vi "CreateCesTML.vi"(8 "error in (no error)":errorcluster, 10 "Traffic String":string="{\"longitude\":-79.645,\"latitude\":39.75710,\"height\":30000,\"ICAO\":\"AAAA\"},{\"longitude\":-79.645,\"latitude\":39.75710,\"height\":5000,\"ICAO\":\"BBBB\"}", 11 "ViewerData":T1={"ViewerLat"="40.286792", "ViewerLong"="-79.541260", "ViewerAlt"="1000", "ViewerHDG"="270", "Viewerpitch"="0"}) -> (0 "error out":errorcluster)   [LabVIEW 2020]
uses:
  <vilib>/Utility/NIReport.llb/Report Type.ctl
  <vilib>/printing/OpenHTMLReport.llb/Open HTML Report in Browser (Refnum).vi
  <vilib>/Utility/NIReport.llb/NI_report.lvclass
  <vilib>/Utility/NIReport.llb/NI_ReportGenerationCore.lvlib
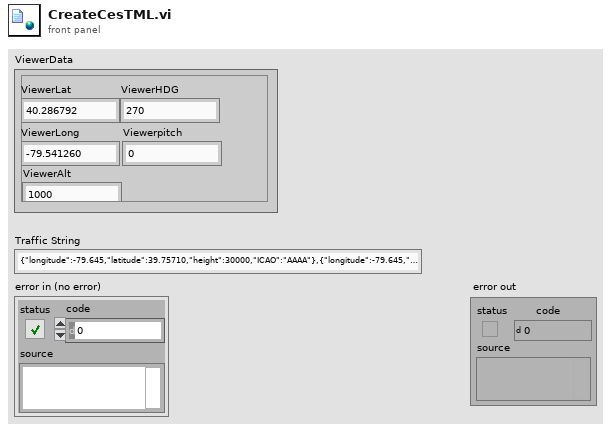
[diagram p1: front panel]
types:
  T1 = cluster{"ViewerLat":string, "ViewerLong":string, "ViewerAlt":string, "ViewerHDG":string, "Viewerpitch":string}
  T2 = typedef "NI_ReportGenerationCore.lvlib/Report Type.ctl" = enum16{"HTML", "Word", "Excel"}
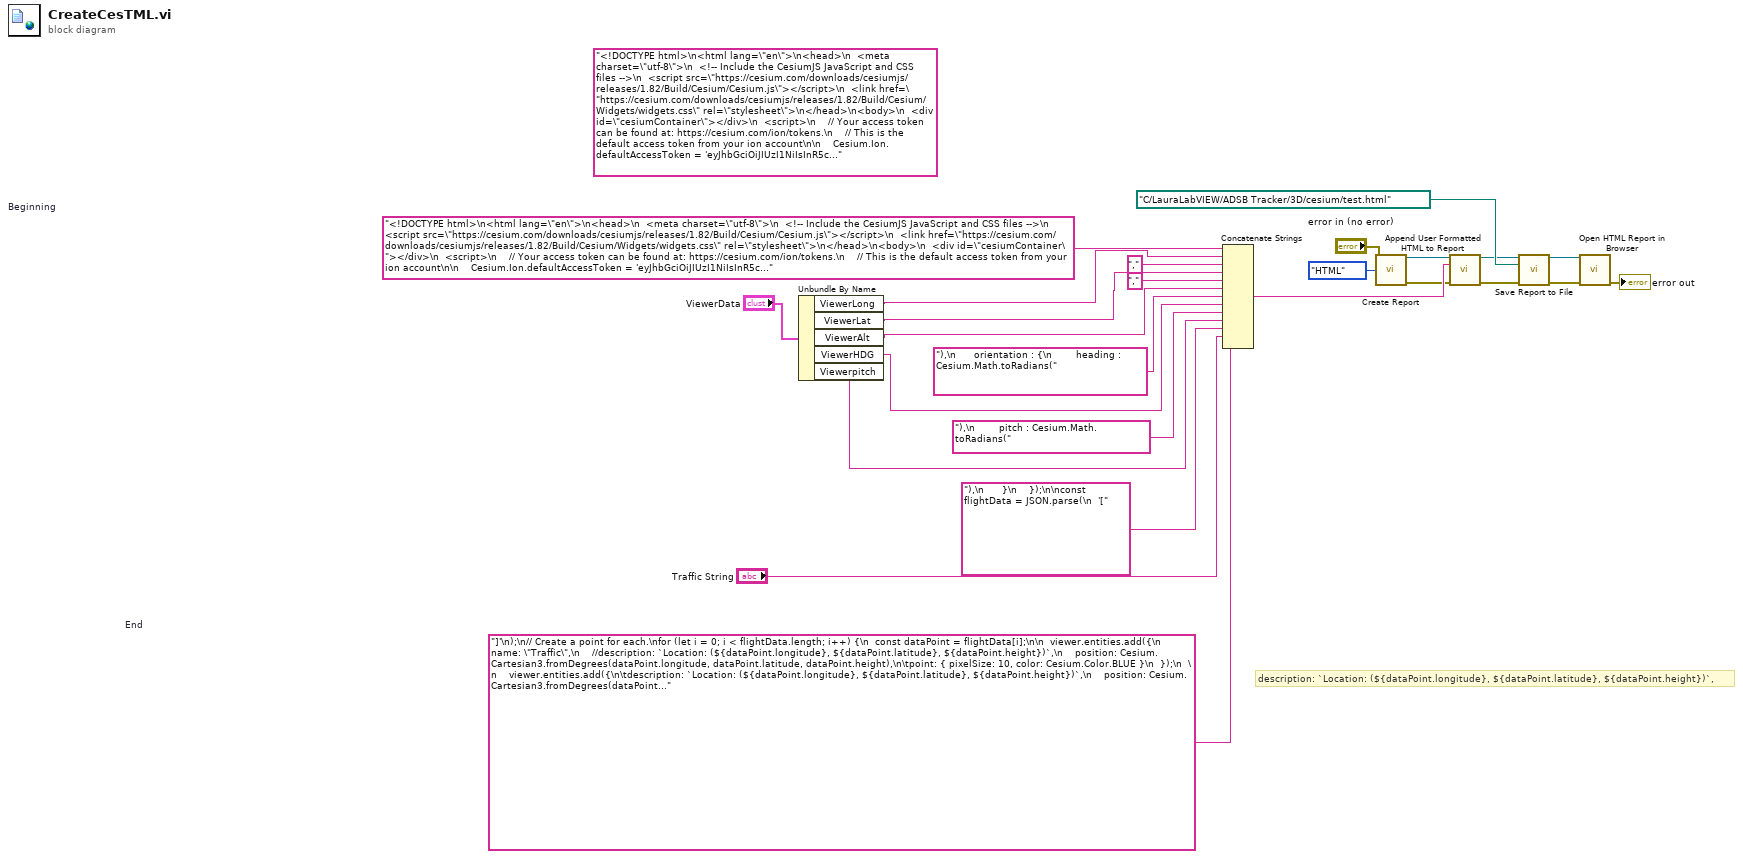
[diagram p0: block diagram]
diagram:
  (unwired) "<!DOCTYPE html>\n<html lang=\"en\">\n<head>\n  <meta charset=\"utf-8\">\n  <!-- Include the CesiumJS JavaScript and CSS files -->\n  <script src=\"https://cesium.com/downloads/cesiumjs/releases/1.82/Build/Cesium/Cesium.js\"></script>\n  <link href=\"https://cesium.com/downloads/cesiumjs/releases/1.82/Build/Cesium/Widgets/widgets.css\" rel=\"stylesheet\">\n</head>\n<body>\n  <div id=\"cesiumContainer\"></div>\n  <script>\n    // Your access token can be found at: https://cesium.com/ion/tokens.\n    // This is the default access token from your ion account\n\n    Cesium.Ion.defaultAccessToken = 'eyJhbGciOiJIUzI1NiIsInR5cCI6IkpXVCJ9.eyJqdGkiOiJmZmNkNjRiZS1hOTkzLTRmNDYtOTM2Mi1iMTFiN2ZmOTk1NzAiLCJpZCI6NjAzMTEsImlhdCI6MTYyNDk3NjYyMX0.UAa42undAhoI0-5rRI83UHZD0L_t9PndA7YpwJBLA6o';\n\t\n\t  // Initialize the Cesium Viewer in the HTML element with the `cesiumContainer` ID.\n    const viewer = new Cesium.Viewer('cesiumContainer', {\n      terrainProvider: Cesium.createWorldTerrain()\n    });    \n    // Add Cesium OSM Buildings, a global 3D buildings layer.\n    const buildingTileset = viewer.scene.primitives.add(Cesium.createOsmBuildings());   \n    // Fly the camera to viewer location\n    viewer.camera.flyTo({\n      destination : Cesium.Cartesian3.fromDegrees(-122.4175, 37.655, 1000),\n      orientation : {\n        heading : Cesium.Math.toRadians(270),\n        pitch : Cesium.Math.toRadians(0),\n      }\n    });\n\nconst flightData = JSON.parse(\n  '[{\"longitude\":-122.39053,\"latitude\":37.61779,\"height\":-27.32},{\"longitude\":-122.39035,\"latitude\":37.61803,\"height\":-27.32}]'\n);\n// Create a point for each.\nfor (let i = 0; i < flightData.length; i++) {\n  const dataPoint = flightData[i];\n\n  viewer.entities.add({\n  name: \"Traffic\",\n    //description: `Location: (${dataPoint.longitude}, ${dataPoint.latitude}, ${dataPoint.height})`,\n    position: Cesium.Cartesian3.fromDegrees(dataPoint.longitude, dataPoint.latitude, dataPoint.height),\n\tpoint: { pixelSize: 10, color: Cesium.Color.BLUE }\n  });\n  \n    viewer.entities.add({\n\tdescription: `Location: (${dataPoint.longitude}, ${dataPoint.latitude}, ${dataPoint.height})`,\n    position: Cesium.Cartesian3.fromDegrees(dataPoint.longitude, dataPoint.latitude, dataPoint.height+50),\n    label: {\n      text: `Location: (${dataPoint.longitude}, ${dataPoint.latitude}, ${dataPoint.height})`,\n\t  font: \"12px Helvetica\",\n\t  pixelOffsetScaleByDistance: new Cesium.NearFarScalar(\n          1.5e2,\n          3.0,\n          1.5e7,\n          0.5\n        ),\n    },\n  });\n  };\n  \n\n  </script>\n </div>\n</body>\n</html>\n\n" ("text to be printed")
  w12 = "]'\n);\n// Create a point for each.\nfor (let i = 0; i < flightData.length; i++) {\n  const dataPoint = flightData[i];\n\n  viewer.entities.add({\n  name: \"Traffic\",\n    //description: `Location: (${dataPoint.longitude}, ${dataPoint.latitude}, ${dataPoint.height})`,\n    position: Cesium.Cartesian3.fromDegrees(dataPoint.longitude, dataPoint.latitude, dataPoint.height),\n\tpoint: { pixelSize: 10, color: Cesium.Color.BLUE }\n  });\n  \n    viewer.entities.add({\n\tdescription: `Location: (${dataPoint.longitude}, ${dataPoint.latitude}, ${dataPoint.height})`,\n    position: Cesium.Cartesian3.fromDegrees(dataPoint.longitude, dataPoint.latitude, dataPoint.height+50),\n    label: {\n      text: `${dataPoint.ICAO} (Long: ${dataPoint.longitude},      Lat: ${dataPoint.latitude}, Alt: ${dataPoint.height}MSL)`,\n\t  font: \"12px Helvetica\",\n\t  pixelOffsetScaleByDistance: new Cesium.NearFarScalar(\n          1.5e2,\n          3.0,\n          1.5e7,\n          0.5\n        ),\n    },\n  });\n  };\n  \n\n  </script>\n </div>\n</body>\n</html>\n\n"  # End
  w23 = "<!DOCTYPE html>\n<html lang=\"en\">\n<head>\n  <meta charset=\"utf-8\">\n  <!-- Include the CesiumJS JavaScript and CSS files -->\n  <script src=\"https://cesium.com/downloads/cesiumjs/releases/1.82/Build/Cesium/Cesium.js\"></script>\n  <link href=\"https://cesium.com/downloads/cesiumjs/releases/1.82/Build/Cesium/Widgets/widgets.css\" rel=\"stylesheet\">\n</head>\n<body>\n  <div id=\"cesiumContainer\"></div>\n  <script>\n    // Your access token can be found at: https://cesium.com/ion/tokens.\n    // This is the default access token from your ion account\n\n    Cesium.Ion.defaultAccessToken = 'eyJhbGciOiJIUzI1NiIsInR5cCI6IkpXVCJ9.eyJqdGkiOiJmZmNkNjRiZS1hOTkzLTRmNDYtOTM2Mi1iMTFiN2ZmOTk1NzAiLCJpZCI6NjAzMTEsImlhdCI6MTYyNDk3NjYyMX0.UAa42undAhoI0-5rRI83UHZD0L_t9PndA7YpwJBLA6o';\n\t\n\t  // Initialize the Cesium Viewer in the HTML element with the `cesiumContainer` ID.\n    const viewer = new Cesium.Viewer('cesiumContainer', {\n      terrainProvider: Cesium.createWorldTerrain()\n    });    \n    // Add Cesium OSM Buildings, a global 3D buildings layer.\n    const buildingTileset = viewer.scene.primitives.add(Cesium.createOsmBuildings());   \n    // Fly the camera to viewer location\n    viewer.camera.flyTo({\n      destination : Cesium.Cartesian3.fromDegrees("  # Beginning
  # "description: `Location: (${dataPoint.longitude}, ${dataPoint.latitude}, ${dataPoint.height})`,"
  n1 = Unbundle By Name("ViewerData") -> ("ViewerLong"=w10:string, "ViewerLat"=w9:string, "ViewerAlt"=w8:string, "ViewerHDG"=w7:string, "Viewerpitch"=w6:string)
  n2 = Concatenate Strings(w23, w10, "," ("string"), w9, "," ("string"), w8, "),\n      orientation : {\n        heading : Cesium.Math.toRadians(" ("concatenated string"), w7, "),\n        pitch : Cesium.Math.toRadians(" ("concatenated string"), w6, "),\n      }\n    });\n\nconst flightData = JSON.parse(\n  '[" ("concatenated string"), "Traffic String", w12) -> (w19:string)
  n3 = call <vilib>:"Create Report.vi"("report type"=Report_Type."HTML", "error in (no error)"="error in (no error)") -> ("report out"=w24:refnum<class "NI_report.lvclass">, "error out"=w4:errorcluster)  [unwired: 12 in]
  n4 = call-dynamic "Append User Formatted HTML to Report.vi"("report in"=w24, "HTML text"=w19, "error in (no error)"=w4) -> ("report out"=w21:refnum<class "NI_report.lvclass">, "error out"=w3:errorcluster)  [unwired: 11 in]
  n5 = call-dynamic "Save Report to File.vi"("report in"=w21, "report file path"=path "C:/LauraLabVIEW/ADSB Tracker/3D/cesium/test.html", "error in (no error)"=w3) -> ("report out"=w20:refnum<class "NI_report.lvclass">, "error out"=w2:errorcluster)  [unwired: 11 in]
  n6 = call-poly <vilib>:"Open HTML Report in Browser.vi"("report in"=w20, "error in (no error)"=w2) -> ("error out"=→"error out":errorcluster)  [unwired: 11 in, 2 out]
